vi "_Test_Main.vi"() -> ()   [LabVIEW 2023, in "LP_CRC.lvlib"]
uses:
  LP_CRC.lvlib
panel:
  out "CRC check":u8=125 format="%x"
  out "size(s)":i32
  in  "String":string
  in  "Frame ID":i32=385 format="%.0x"
  out "CRC calc":u8=125 format="%.0x"
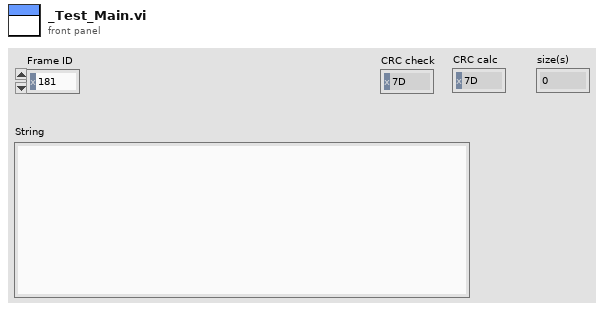
[diagram p1: front panel]
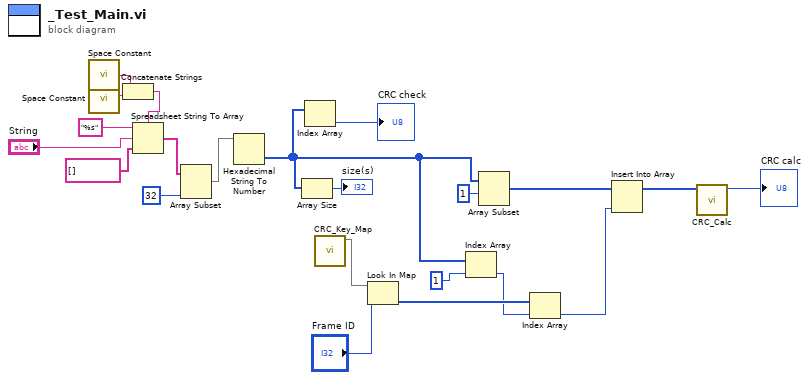
[diagram p0: block diagram]
diagram:
  n1 = call <vilib>:"Space Constant.vi"() -> ("String"=w6:string)
  n2 = call <vilib>:"Space Constant.vi"() -> ("String"=w5:string)
  n3 = Concatenate Strings(w6, w5) -> (w2:string)
  n4 = Spreadsheet String To Array(delimiter (Tab)=w2, format string="%s", spreadsheet string="String", array type (2D Dbl)=string[] []) -> (array=w8:string[])
  n5 = Array Subset(array=w8, length=32) -> (w7:string[])  [unwired: 1 in]
  n6 = Hexadecimal String To Number(string=w7) -> (number=w4:u32[])  [unwired: 2 in, 1 out]
  n7 = Array Size(array=w4) -> (size(s)=→"size(s)":i32)
  n8 = Index Array(array=w4) -> (element=→"CRC check":u32)  [unwired: 1 in]
  n9 = call "CRC_Key_Map.vi"() -> ("Map"=w22:map{i32, u8[]})  [unwired: 11 in]
  n10 = Look In Map(map=w22, key="Frame ID") -> (value=w20:u8[])  [unwired: 1 in, 1 out]
  n11 = Index Array(array=w4, index=1 ("length")) -> (element=w19:u32)
  n12 = Array Subset(array=w4, index=1) -> (w16:u32[])  [unwired: 1 in]
  n13 = Index Array(array=w20, index=w19) -> (element=w15:u8)
  n14 = Insert Into Array(array=w16, new element=w15) -> (w14:u32[])  [unwired: 1 in]
  n15 = call "CRC_Calc.vi"("Data_in"=w14) -> ("CRC"=→"CRC calc":u8)  [unwired: 10 in]
